vi "PQclose.vi"(8 "error in (no error)":errorcluster, 11 "conn":u64) -> (0 "error out":errorcluster)   [LabVIEW 2019, in "libpqutility64.lvlib"]
doc: "Disconnect from PostgreSQL database.\nSee PostgreSQL c-lib doku for further information."
uses:
  libpqutility64.lvlib
  libpqlv64/libpqlv64.lvlib
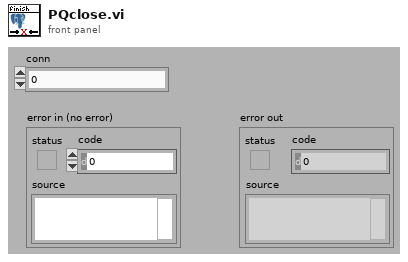
[diagram p1: front panel]
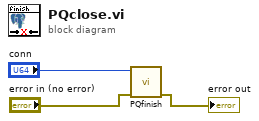
[diagram p0: block diagram]
diagram:
  n1 = call "PQfinish.vi"("error in (no error)"="error in (no error)", "conn"="conn") -> ("error out"=→"error out":errorcluster)  [unwired: 9 in]
